vi "validate.vi"(8 "error in":errorcluster, 11 "TDMS datalogger configuration in":refnum<class "TDMS datalogger configuration.lvclass">) -> (0 "error out":errorcluster, 3 "TDMS datalogger configuration out":refnum<class "TDMS datalogger configuration.lvclass">)   [LabVIEW 2015, in "TDMS datalogger configuration.lvclass"]
doc: "This function performs validation of the configuration. This function should be safe to call at any point and should not rely on anything in the runtime environment."
uses:
  TDMS datalogger configuration.lvclass
  TDMS datalogger configuration.lvclass/TDMS datalogger configuration.ctl
  Read Path.vi
  Read backup directory.vi
  Read log name.vi
  <vilib>/NI/Tag Bus Module Framework/module configuration/TBM module configuration.lvclass
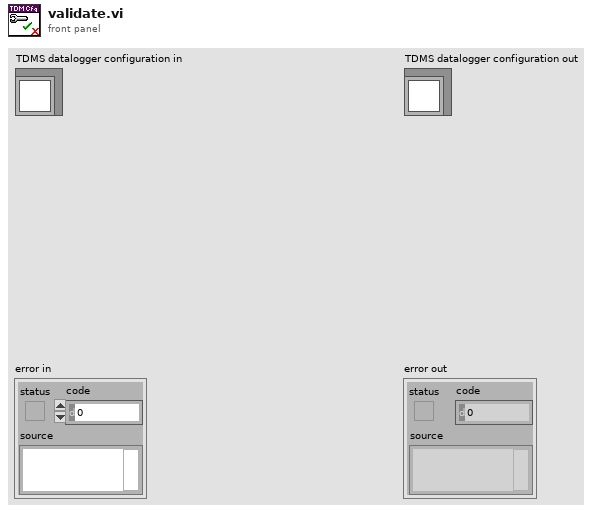
[diagram p1: front panel]
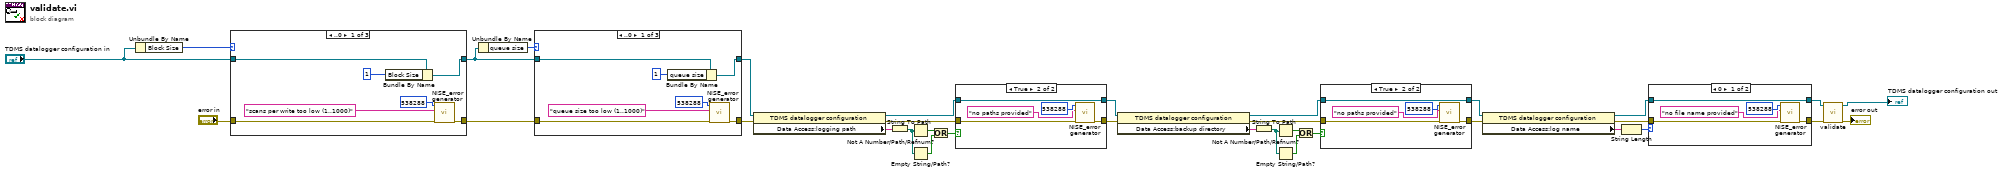
[diagram p0: block diagram]
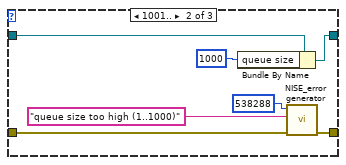
[diagram p4: hidden frame]
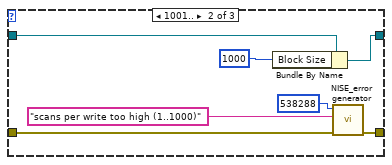
[diagram p6: hidden frame]
diagram:
  n1 = Unbundle By Name("TDMS datalogger configuration in") -> ("Block Size"=w30:u16)
  n2 = case shown="..0" w30 {
    tunnel: [w37 w44 w50] -> w29
    tunnel: "TDMS datalogger configuration in" -> [w38 w45 w50]
    tunnel: [w39 w46 w49] -> w28
    tunnel: "error in" -> [w40 w47 w49]
    frame ..0 {
      n3 = Bundle By Name(cluster=w38, "Block Size"=u16 1 ("scans per write")) -> (w37:refnum<class "TDMS datalogger configuration.lvclass">)
      n4 = call <vilib>:"NISE_error generator.vi"("error in"=w40, "append error message"="scans per write too low (1..1000)" ("error message (\"\")"), "error code (0)"=538288) -> ("error out"=w39:errorcluster)  [unwired: 6 in]
    }
    frame 1001.. {
      n5 = Bundle By Name(cluster=w45, "Block Size"=u16 1000 ("scans per write")) -> (w44:refnum<class "TDMS datalogger configuration.lvclass">)
      n6 = call <vilib>:"NISE_error generator.vi"("error in"=w47, "append error message"="scans per write too high (1..1000)" ("error message (\"\")"), "error code (0)"=538288) -> ("error out"=w46:errorcluster)  [unwired: 6 in]
    }
    frame 1..1000 {
    }
  }
  n7 = Unbundle By Name(w29) -> ("queue size"=w27:u16)
  n8 = case shown="..0" w27 {
    tunnel: [w53 w60 w66] -> w21
    tunnel: w29 -> [w54 w61 w66]
    tunnel: [w55 w62 w65] -> w26
    tunnel: w28 -> [w56 w63 w65]
    frame ..0 {
      n9 = Bundle By Name(cluster=w54, "queue size"=u16 1 ("scans per write")) -> (w53:refnum<class "TDMS datalogger configuration.lvclass">)
      n10 = call <vilib>:"NISE_error generator.vi"("error in"=w56, "append error message"="queue size too low (1..1000)" ("error message (\"\")"), "error code (0)"=538288) -> ("error out"=w55:errorcluster)  [unwired: 6 in]
    }
    frame 1001.. {
      n11 = Bundle By Name(cluster=w61, "queue size"=u16 1000 ("scans per write")) -> (w60:refnum<class "TDMS datalogger configuration.lvclass">)
      n12 = call <vilib>:"NISE_error generator.vi"("error in"=w63, "append error message"="queue size too high (1..1000)" ("error message (\"\")"), "error code (0)"=538288) -> ("error out"=w62:errorcluster)  [unwired: 6 in]
    }
    frame 1..1000 {
    }
  }
  n13 = property class="TDMS datalogger configuration"(reference=w21, error in=w26) -> (reference out=w20:refnum<class "TDMS datalogger configuration.lvclass">, error out=w22:errorcluster, "Data Access:logging path"=w11:string)
  n14 = String To Path(string=w11) -> (path=w10:path)
  n15 = Not A Number/Path/Refnum?(number/path/refnum=w10) -> (NaN/Path/Refnum?=w33:bool)
  n16 = Empty String/Path?(string/path=w10) -> (empty?=w32:bool)
  n17 = Or(x=w33, y=w32) -> (x .or. y?=w31:bool)
  n18 = case shown="True" w31 {
    tunnel: [w68 w72] -> w23
    tunnel: w22 -> [w68 w70]
    tunnel: [w67 w69] -> w18
    tunnel: w20 -> [w67 w69]
    frame False {
    }
    frame True {
      n19 = call <vilib>:"NISE_error generator.vi"("error in"=w70, "append error message"="no paths provided" ("error message (\"\")"), "error code (0)"=538288) -> ("error out"=w72:errorcluster)  [unwired: 6 in]
    }
  }
  n20 = property class="TDMS datalogger configuration"(reference=w18, error in=w23) -> (reference out=w14:refnum<class "TDMS datalogger configuration.lvclass">, error out=w13:errorcluster, "Data Access:backup directory"=w12:string)
  n21 = String To Path(string=w12) -> (path=w9:path)
  n22 = Not A Number/Path/Refnum?(number/path/refnum=w9) -> (NaN/Path/Refnum?=w16:bool)
  n23 = Empty String/Path?(string/path=w9) -> (empty?=w17:bool)
  n24 = Or(x=w16, y=w17) -> (x .or. y?=w15:bool)
  n25 = case shown="True" w15 {
    tunnel: [w75 w77] -> w4
    tunnel: w14 -> [w75 w77]
    tunnel: [w74 w78] -> w3
    tunnel: w13 -> [w74 w76]
    frame False {
    }
    frame True {
      n26 = call <vilib>:"NISE_error generator.vi"("error in"=w76, "append error message"="no paths provided" ("error message (\"\")"), "error code (0)"=538288) -> ("error out"=w78:errorcluster)  [unwired: 6 in]
    }
  }
  n27 = property class="TDMS datalogger configuration"(reference=w4, error in=w3) -> (reference out=w8:refnum<class "TDMS datalogger configuration.lvclass">, error out=w7:errorcluster, "Data Access:log name"=w6:string)
  n28 = String Length(string=w6) -> (length=w5:i32)
  n29 = case shown="0" w5 {
    tunnel: [w84 w87] -> w2
    tunnel: w7 -> [w82 w87]
    tunnel: [w81 w86] -> w1
    tunnel: w8 -> [w81 w86]
    frame 0 {
      n30 = call <vilib>:"NISE_error generator.vi"("error in"=w82, "append error message"="no file name provided" ("error message (\"\")"), "error code (0)"=538288) -> ("error out"=w84:errorcluster)  [unwired: 6 in]
    }
    frame Default {
    }
  }
  n31 = call-parent "validate.vi"("error in"=w2, "configuration in"=w1) -> ("error out"=→"error out":errorcluster, "configuration out"=→"TDMS datalogger configuration out":refnum<class "TDMS datalogger configuration.lvclass">)  [unwired: 8 in]
